vi "Enqueue Previous Picture To Redo.vi"(8 "error in (no error)":errorcluster, 9 "Graphic":refnum<class "Graphic.lvclass">[](array[class]), 10 "Previous Picture":picture, 11 "Canvas in":refnum<class "Canvas.lvclass">) -> (0 "error out":errorcluster, 3 "Canvas out":refnum<class "Canvas.lvclass">)   [LabVIEW 2015, in "Canvas.lvclass"]
uses:
  Canvas.lvclass
  Graphic/Graphic.lvclass
  Canvas.lvclass/Canvas.ctl
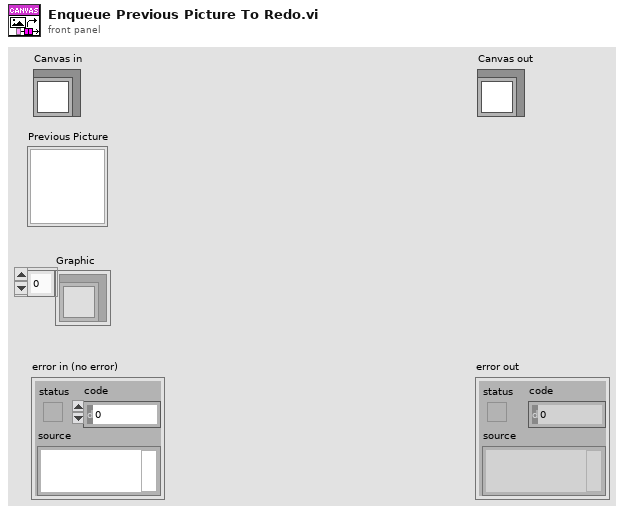
[diagram p1: front panel]
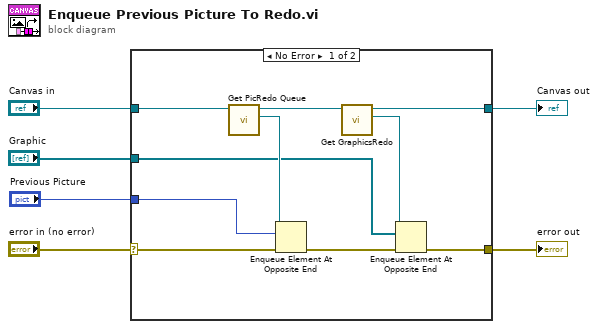
[diagram p0: block diagram]
diagram:
  n1 = case shown="No Error" "error in (no error)" {
    selector: "error in (no error)" -> [w12 w18]
    tunnel: [w8 w18] -> w5
    tunnel: [w11 w17] -> w3
    tunnel: "Canvas in" -> [w16 w17]
    tunnel: "Previous Picture" -> [w13 _]
    tunnel: "Graphic" -> [w7 _]
    frame No Error {
      n2 = call "Get PicRedo Queue.vi"("Canvas in"=w16) -> ("PicRedo Queue"=w14:refnum<queue>, "Canvas out"=w15:refnum<class "Canvas.lvclass">)  [unwired: 8 in, 1 out]
      n3 = Enqueue Element At Opposite End(queue=w14, element=w13, error in (no error)=w12) -> (error out=w10:errorcluster)  [unwired: 1 in, 2 out]
      n4 = call "Get GraphicsRedo.vi"("Canvas in"=w15) -> ("GraphicsRedo"=w9:refnum<queue>, "Canvas out"=w11:refnum<class "Canvas.lvclass">)  [unwired: 8 in, 1 out]
      n5 = Enqueue Element At Opposite End(queue=w9, element=w7, error in (no error)=w10) -> (error out=w8:errorcluster)  [unwired: 1 in, 2 out]
    }
    frame Error {
    }
  }
  "error out" <- w5
  "Canvas out" <- w3
